vi "Change Camera Attributes.vi"(8 "error in":errorcluster, 9 "Object Parameters Attributes":T1={"ReflectedTemperature"=300.0, "AtmosphericTemperature"=300.0, "ExtOpticsTemperature"=300.0, "ObjectEmissivity "=0.95, "RelativeHumidity "=1.0, "ExtOpticsTransmission"=1.0, "EstimatedTransmission"=0.0, "ObjectDistance"=0.0} {"ObjectDistance" min=0.0 max=10000.0 step=1.0; "EstimatedTransmission" min=0.0 max=1.0 step=0.01; "ExtOpticsTransmission" min=0.0 max=1.0 step=0.01; "RelativeHumidity" min=0.0 max=1.0 step=0.01; "ObjectEmissivity" min=0.0 max=1.0 step=0.01; "ExtOpticsTemperature" min=0.0 max=5000.0 step=1.0; "AtmosphericTemperature" min=0.0 max=5000.0 step=1.0; "ReflectedTemperature" min=0.0 max=5000.0 step=1.0}, 10 "Boolean":bool, 11 "Session In":T2) -> (0 "error out":errorcluster, 3 "Session Out":T2)   [LabVIEW 2023]
doc: "Allows the user to change Camera Attributes programatically without restarting the code."
uses:
  <vilib>/userDefined/High Color/IMAQdx.ctl
  <vilib>/vision/driver/NI_Vision_Acquisition_Software.lvlib
  <resource>/objmgr/imaqdx.rc
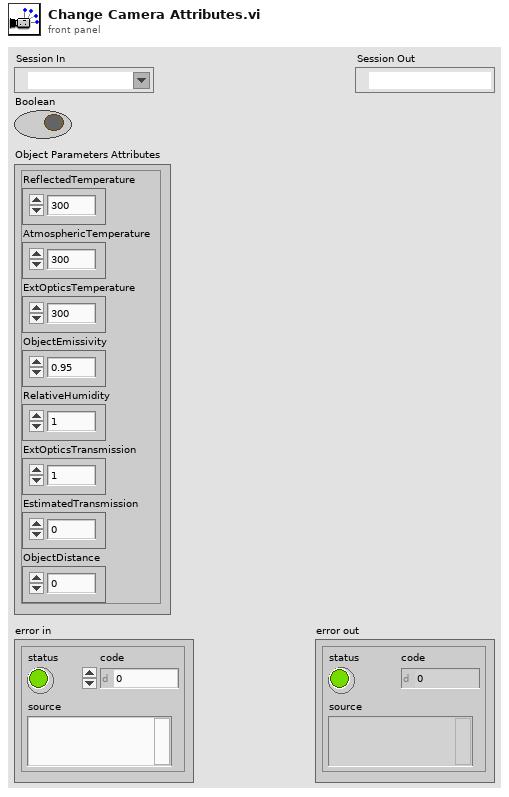
[diagram p1: front panel]
types:
  T1 = cluster{"ReflectedTemperature":dbl, "AtmosphericTemperature":dbl, "ExtOpticsTemperature":dbl, "ObjectEmissivity ":dbl, "RelativeHumidity ":dbl, "ExtOpticsTransmission":dbl, "EstimatedTransmission":dbl, "ObjectDistance":dbl}
  T2 = typedef "IMAQdx.ctl" = refnum<k21>
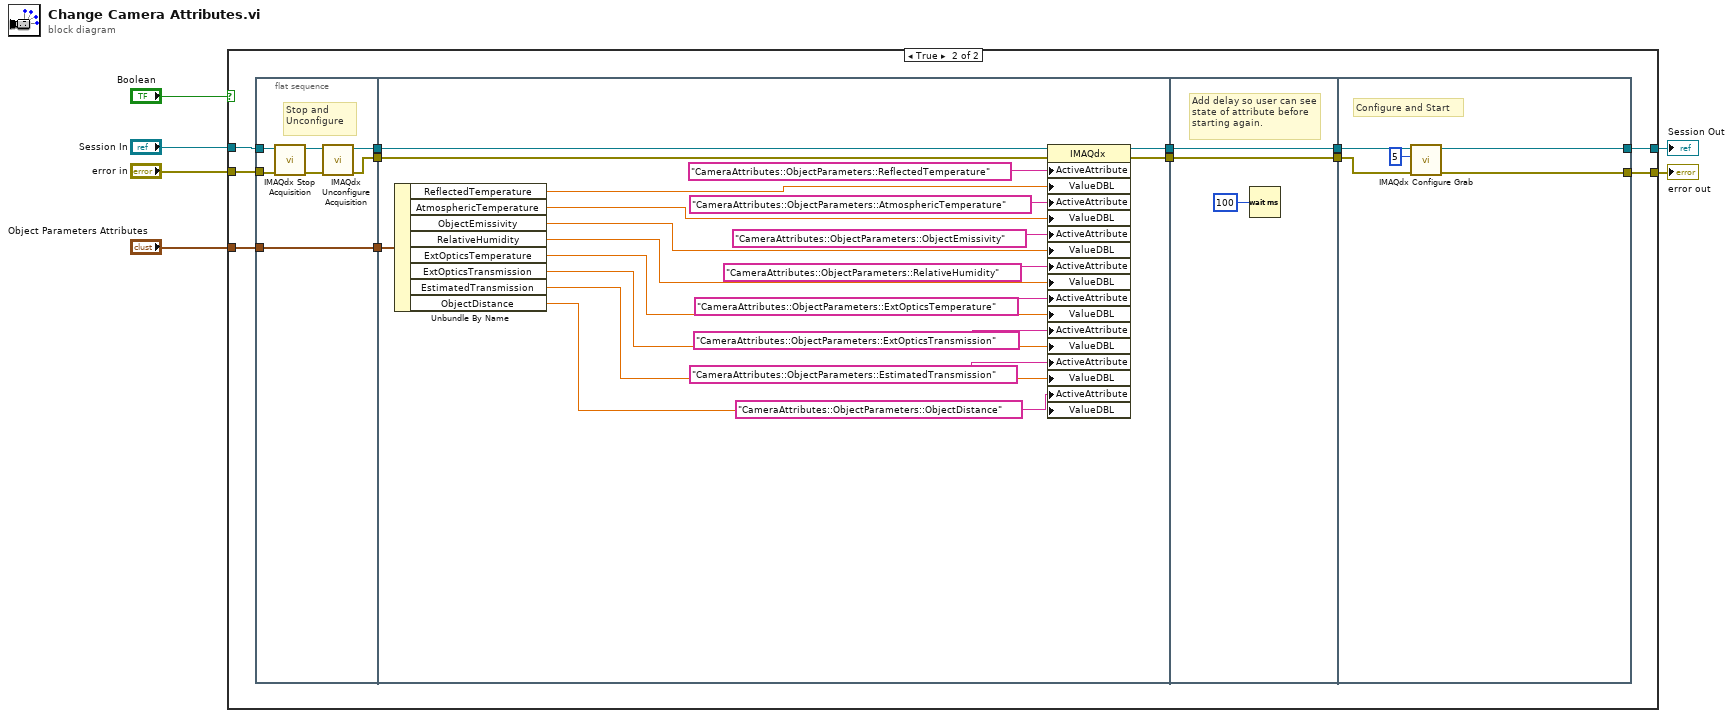
[diagram p0: block diagram]
diagram:
  n1 = case shown="True" "Boolean" {
    tunnel: [w7 w12] -> w2
    tunnel: [w8 w14] -> w3
    tunnel: "Session In" -> [w8 w13]
    tunnel: "error in" -> [w7 w9]
    tunnel: "Object Parameters Attributes" -> [_ w11]
    frame False {
    }
    frame True {
      n2 = flat-sequence {
        tunnel: [w27] -> w20
        tunnel: [w26] -> w19
        tunnel: w13 -> [w23]
        tunnel: w9 -> [w22]
        tunnel: w11 -> [w21]
        tunnel: [w21] -> w10
        tunnel: w20 -> [w48]
        tunnel: w19 -> [w47]
        tunnel: [w46] -> w18
        tunnel: [w45] -> w16
        tunnel: w10 -> [w44]
        tunnel: w18 -> [w51]
        tunnel: [w51] -> w17
        tunnel: w16 -> [w50]
        tunnel: [w50] -> w15
        tunnel: w17 -> [w56]
        tunnel: w15 -> [w55]
        tunnel: [w53] -> w14
        tunnel: [w52] -> w12
        frame #0 {
          # "Stop and Unconfigure"
          n3 = call <vilib>:"IMAQdx Stop Acquisition.vi"("error in"=w22, "Session In"=w23) -> ("error out"=w25:errorcluster, "Session Out"=w24:T2)  [unwired: 8 in]
          n4 = call <vilib>:"IMAQdx Unconfigure Acquisition.vi"("error in"=w25, "Session In"=w24) -> ("error out"=w26:errorcluster, "Session Out"=w27:T2)  [unwired: 8 out]
        }
        frame #1 {
          n5 = Unbundle By Name(w44) -> ("ReflectedTemperature"=w36:dbl, "AtmosphericTemperature"=w35:dbl, "ObjectEmissivity"=w28:dbl, "RelativeHumidity"=w29:dbl, "ExtOpticsTemperature"=w34:dbl, "ExtOpticsTransmission"=w33:dbl, "EstimatedTransmission"=w32:dbl, "ObjectDistance"=w30:dbl)
          n6 = property class="IMAQdx"(reference=w48, error in=w47, "ActiveAttribute"="CameraAttributes::ObjectParameters::ReflectedTemperature", "ValueDBL"=w36, "ActiveAttribute"="CameraAttributes::ObjectParameters::AtmosphericTemperature", "ValueDBL"=w35, "ActiveAttribute"="CameraAttributes::ObjectParameters::ObjectEmissivity", "ValueDBL"=w28, "ActiveAttribute"="CameraAttributes::ObjectParameters::RelativeHumidity", "ValueDBL"=w29, "ActiveAttribute"="CameraAttributes::ObjectParameters::ExtOpticsTemperature", "ValueDBL"=w34, "ActiveAttribute"="CameraAttributes::ObjectParameters::ExtOpticsTransmission", "ValueDBL"=w33, "ActiveAttribute"="CameraAttributes::ObjectParameters::EstimatedTransmission", "ValueDBL"=w32, "ActiveAttribute"="CameraAttributes::ObjectParameters::ObjectDistance", "ValueDBL"=w30) -> (reference out=w46:T2, error out=w45:errorcluster)
        }
        frame #2 {
          # "Add delay so user can see state of attribute before starting again."
          n7 = Wait (ms)(milliseconds to wait=u32 100) -> ()  [unwired: 1 out]
        }
        frame #3 {
          # "Configure and Start"
          n8 = call <vilib>:"IMAQdx Configure Grab.vi"("error in"=w55, "Number of Buffers"=u32 5, "Session In"=w56) -> ("error out"=w52:errorcluster, "Session Out"=w53:T2)  [unwired: 7 in]
        }
      }
    }
  }
  "Session Out" <- w3
  "error out" <- w2
